vi "Setup Position Data.vi"(8 "Error":errorcluster, 9 "FPLocation":T1, 11 "FP":refnum<class "DecFrame_FP.lvclass">) -> (0 "Error Out":errorcluster, 3 "FP Out":refnum<class "DecFrame_FP.lvclass">)   [LabVIEW 2025, in "DecFrame_FP.lvclass"]
uses:
  DecFrame_FP.lvclass
  TypeDefs_Utility/ENUM RB_Pos_Quadrant Position.ctl
  DecFrame_FP.lvclass/DecFrame_FP.ctl
  Frame_FPPos/Frame_FPPos.lvclass
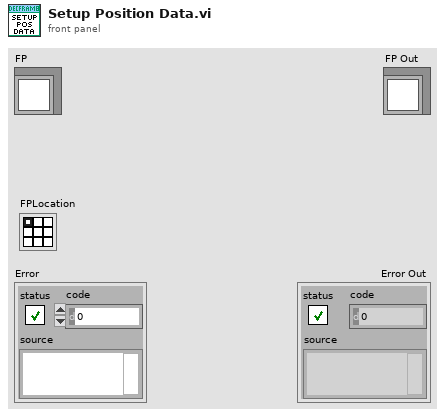
[diagram p1: front panel]
types:
  T1 = typedef "ENUM RB_Pos_Quadrant Position.ctl" = enum32{"LFT-TOP", "MID-TOP", "RGT-TOP", "LFT-CTR", "MID-CTR", "RGT-CTR", "LFT-BOT", "MID-BOT", "RGT-BOT"}
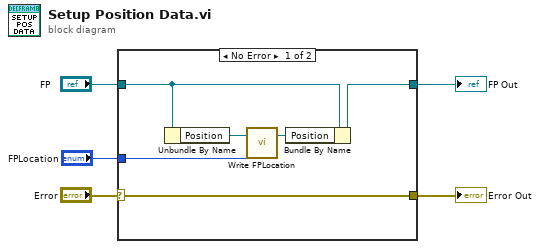
[diagram p0: block diagram]
diagram:
  n1 = case shown="No Error" "Error" {
    selector: "Error" -> [w9 w13]
    tunnel: [w9 w13] -> w4
    tunnel: [w10 w12] -> w2
    tunnel: "FP" -> [w11 w12]
    tunnel: "FPLocation" -> [w6 _]
    frame No Error {
      n2 = Unbundle By Name(w11) -> ("Position"=w8:refnum<class "Frame_FPPos.lvclass">)
      n3 = call "Write FPLocation.vi"("(FPPos)"=w8, "FPLocation"=w6) -> ("(FPPos) Out"=w7:refnum<class "Frame_FPPos.lvclass">)  [unwired: 3 in]
      n4 = Bundle By Name(cluster=w11, "Position"=w7) -> (w10:refnum<class "DecFrame_FP.lvclass">)
    }
    frame Error {
    }
  }
  "Error Out" <- w4
  "FP Out" <- w2
